vi "RampVoltagewithDDSv6,rampgen.vi"(6 "No of samples in ramp":dbl, 7 "Trigger delay NI (ms)":dbl, 9 "Ramp Amplitude (V)}":dbl, 10 "Ramp duration (ms)":dbl, 11 "Plateau duration (ms)":dbl) -> (1 "Numeric 2":i32, 2 "Numeric":dbl, 3 "Sample rate":dbl=500000.0, 4 "Array":dbl[](array[numeric]))   [LabVIEW 2016]
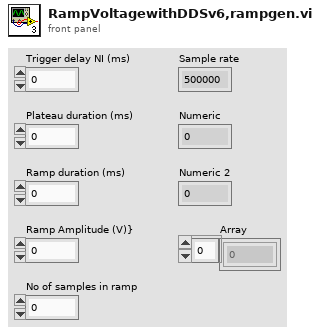
[diagram p1: front panel]
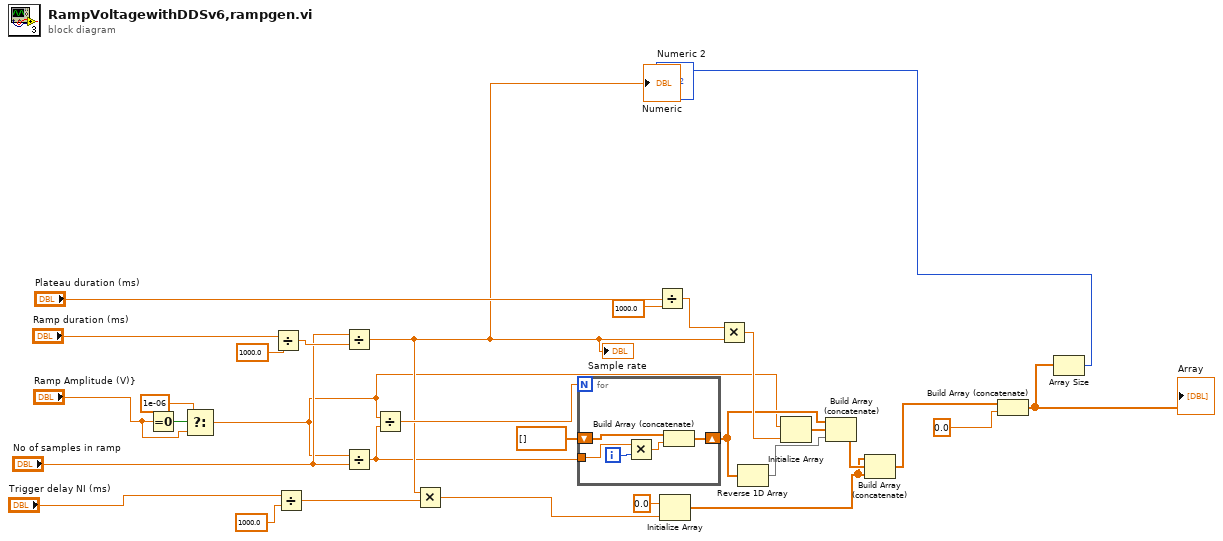
[diagram p0: block diagram]
diagram:
  n1 = Equal To 0?(x="Ramp Amplitude (V)}") -> (x = 0?=w4:bool)
  n2 = Select(t=1e-06, s=w4, f="Ramp Amplitude (V)}") -> (s? t:f=w2:dbl)
  n3 = Divide(x="Ramp duration (ms)", y=1000.0) -> (x/y=w13:dbl)
  n4 = Divide(x="Trigger delay NI (ms)", y=1000.0) -> (x/y=w21:dbl)
  n5 = Divide(x="No of samples in ramp", y=w13) -> (x/y=w22:dbl)
  "Sample rate" <- w22
  "Numeric" <- w22
  n6 = Divide(x=w2, y="No of samples in ramp") -> (x/y=w7:dbl)
  n7 = Divide(x=w2, y=w7) -> (x/y=w24:dbl)
  n8 = Multiply(x=w22, y=w21) -> (x*y=w23:dbl)
  n9 = for {
    N: w24 -> [_]
    shift-right: [w33] -> w8
    shift-left: dbl[] [] -> [w32]
    tunnel: w7 -> [w31]
    i -> [w35]
    n10 = Multiply(x=w31, y=w35) -> (x*y=w34:dbl)
    n11 = Build Array (concatenate)(w32, w34) -> (w33:dbl[])
  }
  n12 = Divide(x="Plateau duration (ms)", y=1000.0) -> (x/y=w15:dbl)
  n13 = Initialize Array(0.0 ("element"), w23) -> (w5:dbl[])
  n14 = Multiply(x=w15, y=w22) -> (x*y=w16:dbl)
  n15 = Reverse 1D Array(array=w8) -> (reversed array=w10:dbl[])
  n16 = Initialize Array(w2, w16) -> (w9:dbl[])
  n17 = Build Array (concatenate)(w8, w9, w10) -> (w18:dbl[])
  n18 = Build Array (concatenate)(w5, w18, w5) -> (w27:dbl[])
  n19 = Build Array (concatenate)(w27, 0.0 ("y")) -> (w30:dbl[])
  "Array" <- w30
  n20 = Array Size(array=w30) -> (size(s)=→"Numeric 2":i32)
